vi "Funct TIFF export-Experiment folder validator.vi"(8 "error in (no error)":errorcluster) -> (0 "error out":errorcluster, 2 "Valid experiment folders found":bool, 3 "Filtered Array out":path[](array[path]))   [LabVIEW 2020]
uses:
  Globals/gl_funct TIFF export globals.vi
  <userlib>/_OpenG.lib/array/array.llb/Conditional Auto-Indexing Tunnel (Path)__ogtk.vi
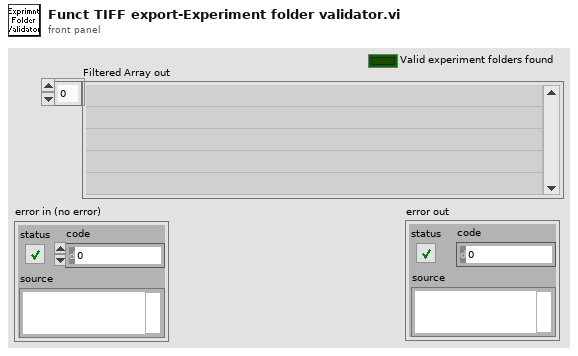
[diagram p1: front panel]
types:
  T1 = typedef "Funct TIFF exporter ctrl refs.ctl" = cluster{"This VI":refnum<vi>, "Current Experiment":refnum<vi>, "Imaging protocol":refnum<vi>, "Predominant ROI type":refnum<vi>, "Patches in Experiment":refnum<vi>, "Folder Path":refnum<vi>, "Export":refnum<vi>, "Trial number":refnum<vi>, "Output TIFF type":refnum<vi>}
  T2 = typedef "Fixed strings.ctl" = cluster{"ROI file name":string, "Normalised ROI file name":string, "Zplane Pockels values file name":string, "Functional data folder name":string, "Experiment Header file name":string, "Z-stack images folder name":string, "Groups setup rel. path":string, "Groups text file rel. path":string, "TDMS files folder name (F.img)":string, "TDMS files folder name (V.acq)":string, "TDMS files folder name (Pl.acq)":string, "Cycle rel times sequence file":string, "Dynamically called VIs folder name":string, "Time Series folder base name":string}
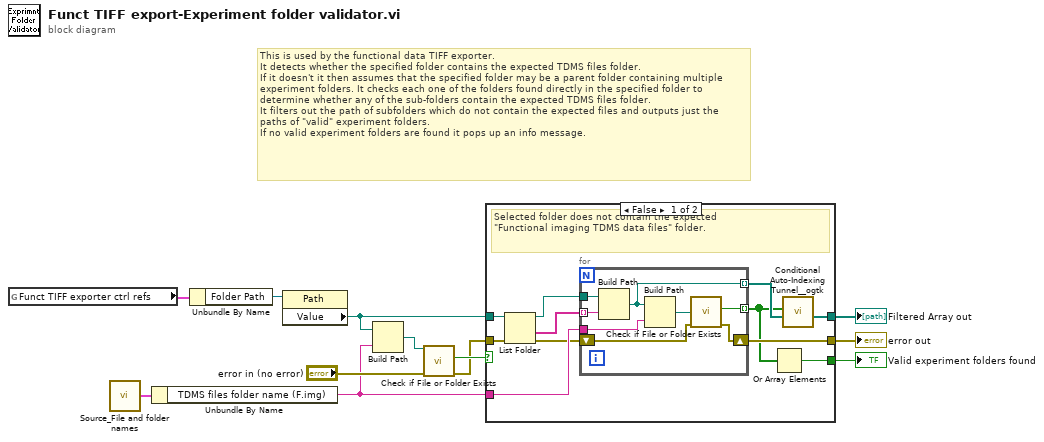
[diagram p0: block diagram]
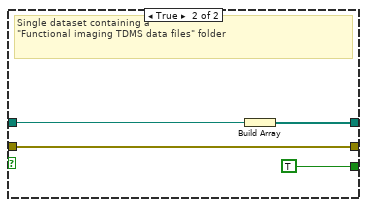
[diagram p2: hidden frame]
diagram:
  # "This is used by the functional data TIFF exporter.\nIt detects whether the specified folder contains the expected TDMS files folder.\nIf it doesn't it then assumes that the specified folder may be a parent folder containing multiple experiment folders. It checks each one of the folders found directly in the specified folder to determine whether any of the sub-folders contain the expected TDMS files folder.\nIt filters out the path of subfolders which do not contain the expected files and outputs just the paths of \"valid\" experiment folders.\nIf no valid experiment folders are found it pops up an info message."
  n1 = global read "gl_funct TIFF export globals.vi" "Funct TIFF exporter ctrl refs"() -> (w10:T1)
  n2 = call "Source_File and folder names.vi"() -> ("Fixed strings"=w2:T2)  [unwired: 1 in]
  n3 = Unbundle By Name(w2) -> ("TDMS files folder name (F.img)"=w1:string)
  n4 = Unbundle By Name(w10) -> ("Folder Path"=w3:refnum<vi>)
  n5 = property on="Property Node" class="Path"(reference=w3) -> ("Value"=w6:path)  [unwired: 1 in, 2 out]
  n6 = Build Path(base path=w6, name or relative path=w1) -> (appended path=w5:path)
  n7 = call <vilib>:"Check if File or Folder Exists.vi"("error in (no error)"="error in (no error)", "path"=w5) -> ("error out"=w8:errorcluster, "file or folder exists?"=w9:bool)  [unwired: 7 in, 1 out]
  n8 = case shown="False" w9 {
    tunnel: w6 -> [w23 w34]
    tunnel: [w17 w33] -> w11
    tunnel: w8 -> [w22 w35]
    tunnel: [w15 w35] -> w4
    tunnel: w1 -> [w21 _]
    tunnel: [w13 TRUE] -> w12
    frame False {
      # "Selected folder does not contain the expected\n\"Functional imaging TDMS data files\" folder."
      n9 = List Folder(path=w23, error in=w22) -> (path out=w18:path, folder names=w20:string[], error out=w16:errorcluster)  [unwired: 2 in, 1 out]
      n10 = for {
        tunnel: w20 -> [w30] mode=indexing
        tunnel: w18 -> [w31]
        tunnel: w21 -> [w29]
        tunnel: [w27] -> w14 mode=indexing
        tunnel: [w26] -> w19 mode=indexing
        shift-right: [w24] -> w15
        shift-left: w16 -> [w25]
        n11 = Build Path(base path=w31, name or relative path=w30) -> (appended path=w26:path)
        n12 = Build Path(base path=w26, name or relative path=w29) -> (appended path=w28:path)
        n13 = call <vilib>:"Check if File or Folder Exists.vi"("error in (no error)"=w25, "path"=w28) -> ("error out"=w24:errorcluster, "file or folder exists?"=w27:bool)  [unwired: 7 in, 1 out]
      }
      n14 = Or Array Elements(Boolean array=w14) -> (logical OR=w13:bool)
      n15 = call-poly <userlib>:"Conditional Auto-Indexing Tunnel__ogtk.vi"("Array in"=w19, "Elements to keep"=w14) -> ("Filtered Array out"=w17:path[])  [unwired: 5 in]
    }
    frame True {
      # "Single dataset containing a\n\"Functional imaging TDMS data files\" folder"
      n16 = Build Array(w34) -> (w33:path[])
    }
  }
  "Valid experiment folders found" <- w12
  "Filtered Array out" <- w11
  "error out" <- w4
